vi "Acquire_Spatial.vi"(8 "error in (no error)":errorcluster, 11 "FROG in":refnum<class "FROG.lvclass">) -> (0 "error out":errorcluster, 3 "frogTrace":T1)   [LabVIEW 2020, in "FROG.lvclass"]
uses:
  FROG.lvclass
  <vilib>/vision/Image Controls.llb/IMAQ Image.ctl
  FROG.lvclass/FROG.ctl
  Point Grey Camera/GUIcompressionCluster.ctl
  shared/OnOffTypeDef.ctl
  <userlib>/_OpenG.lib/error/error.llb/Filter Error Codes (Array)__ogtk.vi
  shared/CompressAndUpdate(Poly)/CompressAndUpdate(IMAQ Image).vi
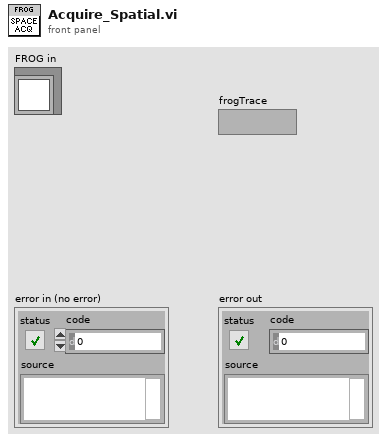
[diagram p1: front panel]
types:
  T1 = typedef "IMAQ Image.ctl" = refnum<image>
  T2 = typedef "OnOffTypeDef.ctl" = enum16{"off", "on"}
  T3 = typedef "GUIcompressionCluster.ctl" = cluster{"GUI8bit":T2, "GUICompression":T2, "CompressionQuality":i32}
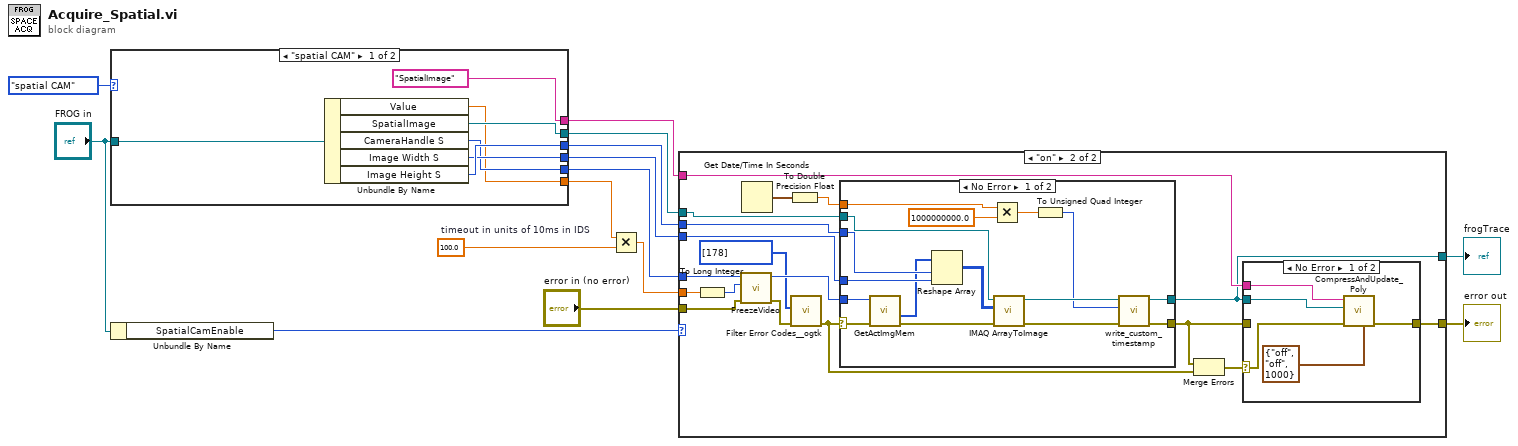
[diagram p0: block diagram]
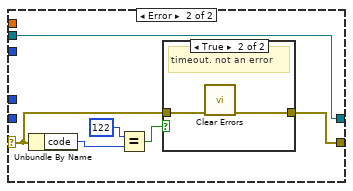
[diagram p4: hidden frame]
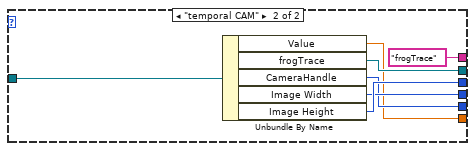
[diagram p6: hidden frame]
diagram:
  w6 = 100.0  # timeout in units of 10ms in IDS
  n1 = case shown="\"spatial CAM\"" enum16{"temporal CAM", "spatial CAM"}."spatial CAM" ("cameraselect") {
    tunnel: [w21 w28] -> w10
    tunnel: [w20 w27] -> w9
    tunnel: [w19 w26] -> w8
    tunnel: [w18 w25] -> w7
    tunnel: [w17 w24] -> w5
    tunnel: "FROG in" -> [w16 w23]
    tunnel: ["SpatialImage" ("command or variable name") "frogTrace" ("command or variable name")] -> w3
    frame "spatial CAM" {
      n2 = Unbundle By Name ("pressure read")(w16) -> ("Value"=w17:dbl, "SpatialImage"=w21:T1, "CameraHandle S"=w18:u32, "Image Width S"=w19:i32, "Image Height S"=w20:i32)
    }
    frame "temporal CAM" {
      n3 = Unbundle By Name ("pressure read")(w23) -> ("Value"=w24:dbl, "frogTrace"=w28:T1, "CameraHandle"=w25:u32, "Image Width"=w26:i32, "Image Height"=w27:i32)
    }
  }
  n4 = Unbundle By Name("FROG in") -> ("SpatialCamEnable"=w1:T2)
  n5 = Multiply(x=w5, y=w6) -> (x*y=w4:dbl)
  n6 = case shown="\"on\"" w1 {
    tunnel: w3 -> [_ w48]
    tunnel: w4 -> [_ w44]
    tunnel: w7 -> [_ w42]
    tunnel: w8 -> [_ w41]
    tunnel: w9 -> [_ w40]
    tunnel: w10 -> [w30 w39]
    tunnel: "error in (no error)" -> [w29 w38]
    tunnel: [w29 w37] -> w13
    tunnel: [w30 w34] -> w14
    frame "off", Default {
    }
    frame "on" {
      n7 = To Long Integer(number=w44) -> (32bit integer=w43:i32)
      n8 = call "FreezeVideo.vi"("error in"=w38, "Wait"=w43, "Camera Handle In"=w42) -> ("error out"=w36:errorcluster, "Camera Handle Out"=w45:u32)  [unwired: 7 out]
      n9 = Get Date/Time In Seconds() -> (seconds since 1Jan1904=w32:timestamp)
      n10 = To Double Precision Float(number=w32) -> (double precision float=w31:dbl)
      n11 = call-poly <userlib>:"Filter Error Codes__ogtk.vi"("Error In"=w36, "Error Codes to Filter"=i32[] [178]) -> ("Error Out"=w35:errorcluster)  [unwired: 7 in, 2 out]
      n12 = case shown="No Error" w35 {
        selector: w35 -> [w63 w71]
        tunnel: w39 -> [w70 w73]
        tunnel: w41 -> [w69 _]
        tunnel: w40 -> [w68 _]
        tunnel: w45 -> [w66 _]
        tunnel: [w59 w72] -> w47
        tunnel: [w61 w73] -> w34
        tunnel: w31 -> [w55 _]
        frame No Error {
          n13 = call "GetActImgMem.vi"("error in"=w63, "Camera Handle In"=w66) -> ("error out"=w67:errorcluster, "Image Memory Out"=w65:u8[])  [unwired: 8 out]
          n14 = Reshape Array(w65, w68, w69) -> (w64:u8[][])
          n15 = Multiply(x=w55, y=1000000000.0) -> (x*y=w57:dbl)
          n16 = call "IMAQ ArrayToImage"("error in (no error)"=w67, "Image Pixels (U8)"=w64, "Image"=w70) -> ("error out"=w60:errorcluster, "Image Out"=w62:T1)  [unwired: 7 in]
          n17 = To Unsigned Quad Integer(1:w57) -> (0:w56:u64)
          n18 = call "write_custom_timestamp.vi"("error in (no error)"=w60, "timestamp (ns)"=w56, "Refnum in"=w62) -> ("error out"=w59:errorcluster, "Refnum out"=w61:T1)  [unwired: 7 in]
        }
        frame Error {
          n19 = Unbundle By Name(w71) -> ("code"=w76:i32)
          n20 = Equal?(x=122, y=w76) -> (x = y?=w74:bool)
          n21 = case shown="True" w74 {
            tunnel: w71 -> [w77 w79]
            tunnel: [w77 w78] -> w72
            frame False {
            }
            frame True {
              # "timeout. not an error"
              n22 = call <vilib>:"Clear Errors.vi"("error in (no error)"=w79) -> ("error out"=w78:errorcluster)  [unwired: 5 in, 1 out]
            }
          }
        }
      }
      n23 = Merge Errors(w47, w35) -> (w46:errorcluster)
      n24 = case shown="No Error" w46 {
        selector: w46 -> [w50 _]
        tunnel: [w51 w54] -> w37
        tunnel: w34 -> [w52 _]
        tunnel: w47 -> [_ w54]
        tunnel: w48 -> [w49 _]
        frame No Error {
          n25 = call-poly "CompressAndUpdate_Poly.vi"("GUICompression"=T3 {"GUI8bit"=enum."off", "GUICompression"=enum."off", "CompressionQuality"=1000}, "error in"=w50, "IMAQ Image"=w52, "command or variable name"=w49) -> ("error out"=w51:errorcluster)  [unwired: 7 in]
        }
        frame Error {
        }
      }
    }
  }
  "frogTrace" <- w14
  "error out" <- w13
